vi "ArduinoCoreService.vi"() -> ()   [LabVIEW 2023]
uses:
  <vilib>/MakerHub/LINX/Public/Peripherals/Digital/Digital Write 1 Chan.vi
  <vilib>/MakerHub/LINX/Public/Peripherals/Digital/Digital Write N Chans.vi
  <vilib>/MakerHub/LINX/Private/Local IO/LinxDigitalWrite.vi
  <vilib>/MakerHub/LINX/Public/Utilities/Check Channel.vi
  <vilib>/MakerHub/LINX/Public/Utilities/Open Serial.vi
  PinoutSettings.vi
  Actuators.vi
  <vilib>/MakerHub/LINX/Private/Utilties/Generate Error.vi
  <vilib>/MakerHub/LINX/Public/Sensors/Temperature/TMP3x/TMP36.vi
  Sensors.vi
  <vilib>/MakerHub/LINX/LMH-LINX.lvlib
  <vilib>/MakerHub/LINX/Public/Sensors/Temperature/TMP3x/TMP3x.lvlib
  <vilib>/MakerHub/LINX/Public/Sensors/Distance/Ultrasonic/Ultrasonic.lvlib
panel:
  out "Centimeters":dbl
  in  "Serial Port":refnum<visa-resource-name>="N/A"
  in  "Stop Button":bool
  out "Loop Rate (Hz)":u32
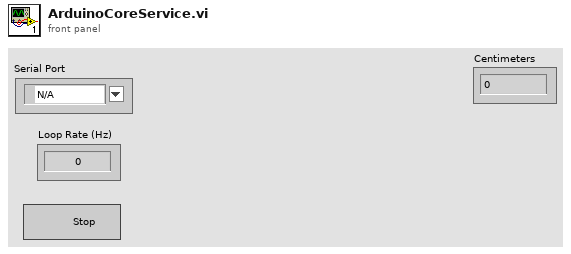
[diagram p1: front panel]
types:
  T1 = typedef "LMH-LINX.lvlib/LINX Ref.ctl" = cluster{"IO":T2, "Interface":T3, "LINX Device Config":T4}
  T2 = typedef "LMH-LINX.lvlib/Platform.ctl" = enum16{"Remote", "Local"}
  T3 = typedef "LMH-LINX.lvlib/Interface.ctl" = enum16{"Serial", "TCP"}
  T4 = typedef "LMH-LINX.lvlib/Device.lvlib/LINX Device Config.ctl" = cluster{"Interface":T3, "COM Port":refnum<visa-resource-name>, "TCP Configuration":T5, "Device Family":u8, "Device ID":u8, "Device Name":string, "TCP Ref":refnum<k5>, "Channels":T6}
  T5 = typedef "LMH-LINX.lvlib/Device.lvlib/TCP Config.ctl" = cluster{"IP Address":string, "Port":u16}
  T6 = typedef "LMH-LINX.lvlib/Channels.ctl" = cluster{"DI":u8[], "DO":u8[], "AI":u8[], "AO":u8[], "PWM":u8[], "QE":u8[], "UART":u8[], "I2C 2":u8[], "SPI":u8[], "CAN":u8[], "Servo":u8[], "AI Ref (V)":dbl, "AI Resolution (Bits)":u8, "AO Ref (V)":dbl, "AO Resolution (Bits)":u8}
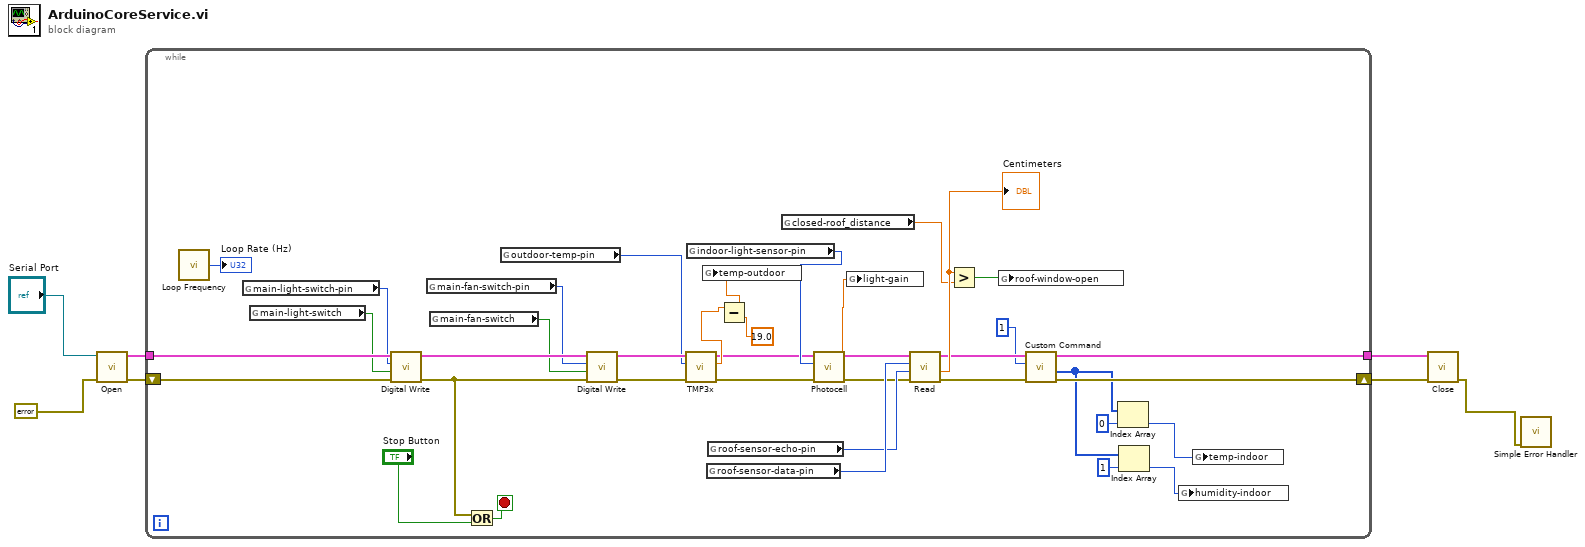
[diagram p0: block diagram]
diagram:
  n1 = call-poly <vilib>:"Open.vi"("Error In"=errorcluster {"status"=FALSE, "code"=0, "source"=""}, "Serial Port"="Serial Port") -> ("Error Out"=w6:errorcluster, "LINX Resource"=w7:T1)  [unwired: 7 in, 1 out]
  n2 = while {
    tunnel: w7 -> [w43]
    tunnel: [w14] -> w5
    shift-right: [w16] -> w4
    shift-left: w6 -> [w42]
    stop <- w45 stop-if-true
    n3 = call <vilib>:"Loop Frequency.vi"() -> ("Loop Rate (Hz)"=→"Loop Rate (Hz)":u32)
    n4 = global read "PinoutSettings.vi" "main-light-switch-pin"() -> (w40:u8)
    n5 = global read "Actuators.vi" "main-light-switch"() -> (w39:bool)
    n6 = call-poly <vilib>:"Digital Write.vi"("Error In"=w42, "Output Value"=w39, "DO Channel"=w40, "LINX Resource"=w43) -> ("Error Out"=w37:errorcluster, "LINX Resource"=w38:T1)  [unwired: 6 in]
    n7 = global read "PinoutSettings.vi" "main-fan-switch-pin"() -> (w36:u8)
    n8 = global read "Actuators.vi" "main-fan-switch"() -> (w35:bool)
    n9 = Or(x=w37, y="Stop Button") -> (x .or. y?=w45:bool)
    n10 = global read "PinoutSettings.vi" "outdoor-temp-pin"() -> (w32:u8)
    n11 = call-poly <vilib>:"Digital Write.vi"("Error In"=w37, "Output Value"=w35, "DO Channel"=w36, "LINX Resource"=w38) -> ("Error Out"=w33:errorcluster, "LINX Resource"=w34:T1)  [unwired: 6 in]
    n12 = call-poly <vilib>:"TMP3x.vi"("Error In"=w33, "Analog Channel"=w32, "LINX Resource"=w34) -> ("Error Out"=w21:errorcluster, "Temp C"=w25:dbl, "LINX Resource"=w20:T1)  [unwired: 6 in]
    n13 = global read "PinoutSettings.vi" "indoor-light-sensor-pin"() -> (w23:u8)
    n14 = global read "PinoutSettings.vi" "roof-sensor-data-pin"() -> (w28:u8)
    n15 = global read "PinoutSettings.vi" "roof-sensor-echo-pin"() -> (w27:u8)
    n16 = Subtract(x=w25, y=19.0) -> (x-y=w26:dbl)
    n17 = global write "Sensors.vi" "temp-outdoor"(w26) -> ()
    n18 = global read "PinoutSettings.vi" "closed-roof_distance"() -> (w29:dbl)
    n19 = call <vilib>:"Photocell.vi"("Error In"=w21, "AI Channel"=w23, "LINX Resource"=w20) -> ("Error Out"=w22:errorcluster, "Value (0-100)"=w18:dbl, "LINX Resource"=w19:T1)  [unwired: 6 in]
    n20 = global write "Sensors.vi" "light-gain"(w18) -> ()
    n21 = call <vilib>:"Read.vi"("Error In"=w22, "DO Channel"=w27, "DI Channel"=w28, "LINX Resource"=w19) -> ("Error Out"=w17:errorcluster, "Centimeters"=w30:dbl, "LINX Resource"=w15:T1)  [unwired: 4 in, 1 out]
    "Centimeters" <- w30
    n22 = Greater?(x=w30, y=w29) -> (0:w31:bool)
    n23 = global write "Sensors.vi" "roof-window-open"(w31) -> ()
    n24 = call <vilib>:"Custom Command.vi"("Error In"=w17, "Custom Command Number"=u16 1, "LINX Resource"=w15) -> ("Error Out"=w16:errorcluster, "Response"=w11:u8[], "LINX Resource"=w14:T1)  [unwired: 5 in, 1 out]
    n25 = Index Array(array=w11, index=0) -> (element=w9:u8)
    n26 = Index Array(array=w11, index=1) -> (element=w8:u8)
    n27 = global write "Sensors.vi" "humidity-indoor"(w8) -> ()
    n28 = global write "Sensors.vi" "temp-indoor"(w9) -> ()
  }
  n29 = call <vilib>:"Close.vi"("Error In"=w4, "LINX Resource"=w5) -> ("Error Out"=w3:errorcluster)  [unwired: 9 in]
  n30 = call <vilib>:"Simple Error Handler.vi"("error in (no error)"=w3) -> ()  [unwired: 4 in, 5 out]
